vi "Get Enqueuer from Tag.vi"(10 "Tag":string) -> (2 "Enqueuer":refnum<class "Message Enqueuer.lvclass">)   [LabVIEW 2023, in "Monitored Actor.lvlib" / "Classic Monitor.lvclass"]
doc: "Converst the tree tag to an enqueuer object\n\nCopyright: MGI 2016\nAuthor: Derek Trepanier"
uses:
  Classic Monitor.lvclass
  builds/Framework/Actor Framework.lvlibp/1abvi3w/vi.lib/ActorFramework/Message Enqueuer/Message Enqueuer.lvclass
  Classic Monitor.lvclass/Classic Monitor.ctl
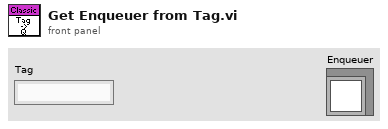
[diagram p1: front panel]
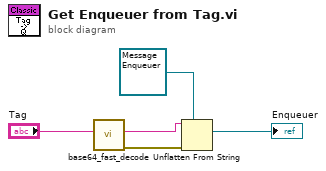
[diagram p0: block diagram]
diagram:
  n1 = call "base64_fast_decode.vi"("string in (base64-encoded)"="Tag") -> ("error out"=w3:errorcluster, "string out (decoded)"=w4:string)  [unwired: 9 in]
  n2 = Unflatten From String(type=refnum<class "Message Enqueuer.lvclass"> refnum ("Enqueuer"), binary string=w4, error in (no error)=w3) -> (value=→"Enqueuer":refnum<class "Message Enqueuer.lvclass">)  [unwired: 2 in, 2 out]
